vi "Add Subscription.vi"(8 "error in (no error)":errorcluster, 9 "SessionMailbox":refnum<queue>, 10 "Topic Subscription":T1, 11 "MQTT_Base in":refnum<class "MQTT_Base.lvclass">) -> (0 "error out":errorcluster, 1 "Failed":bool, 3 "MQTT_Base out":refnum<class "MQTT_Base.lvclass">)   [LabVIEW 2013, in "MQTT Base.lvlib" / "MQTT_Base.lvclass"]
uses:
  MQTT_Base.lvclass
  <vilib>/LabVIEW Open Source Project/MQTT Control Packets/Control Packets/SUBSCRIBE/Topic Subscription -- cluster.ctl
  <vilib>/LabVIEW Open Source Project/MQTT Control Packets/Control Packets/ControlPacket/QualityOfService -- enum.ctl
  Response -- cluster.ctl
  <vilib>/LabVIEW Open Source Project/MQTT Control Packets/Control Packets/ControlPacket/ControlPacket.lvclass
  MQTT_Base.lvclass/MQTT_Base.ctl
  Subscription/Subscription.lvclass/Subscription.ctl
  TopicFilter/TopicFilter.lvclass/TopicFilter.ctl
  Subscription/Subscription.lvclass
  <vilib>/LabVIEW Open Source Project/MQTT Control Packets/Control Packets/SUBSCRIBE/SUBSCRIBE.lvclass
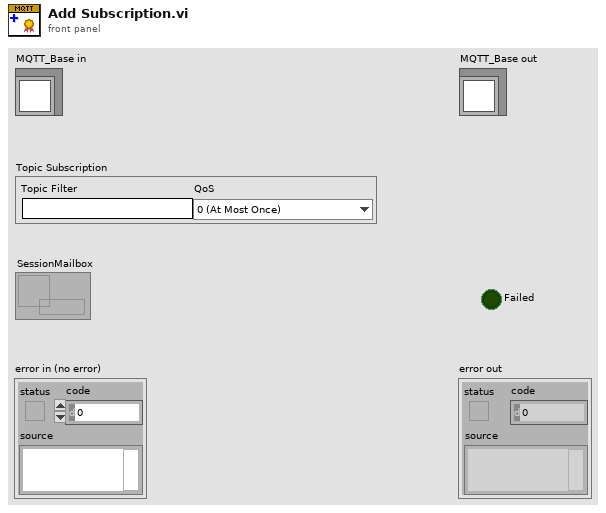
[diagram p1: front panel]
types:
  T1 = typedef "MQTT_Control_Packets.lvlib/SUBSCRIBE.lvclass/Topic Subscription -- cluster.ctl" = cluster{"Topic Filter":string, "QoS":T2}
  T2 = typedef "MQTT_Control_Packets.lvlib/ControlPacket.lvclass/QualityOfService -- enum.ctl" = enum16{"0 (At Most Once)", "1 (At Least Once)", "2 (Exactly Once)"}
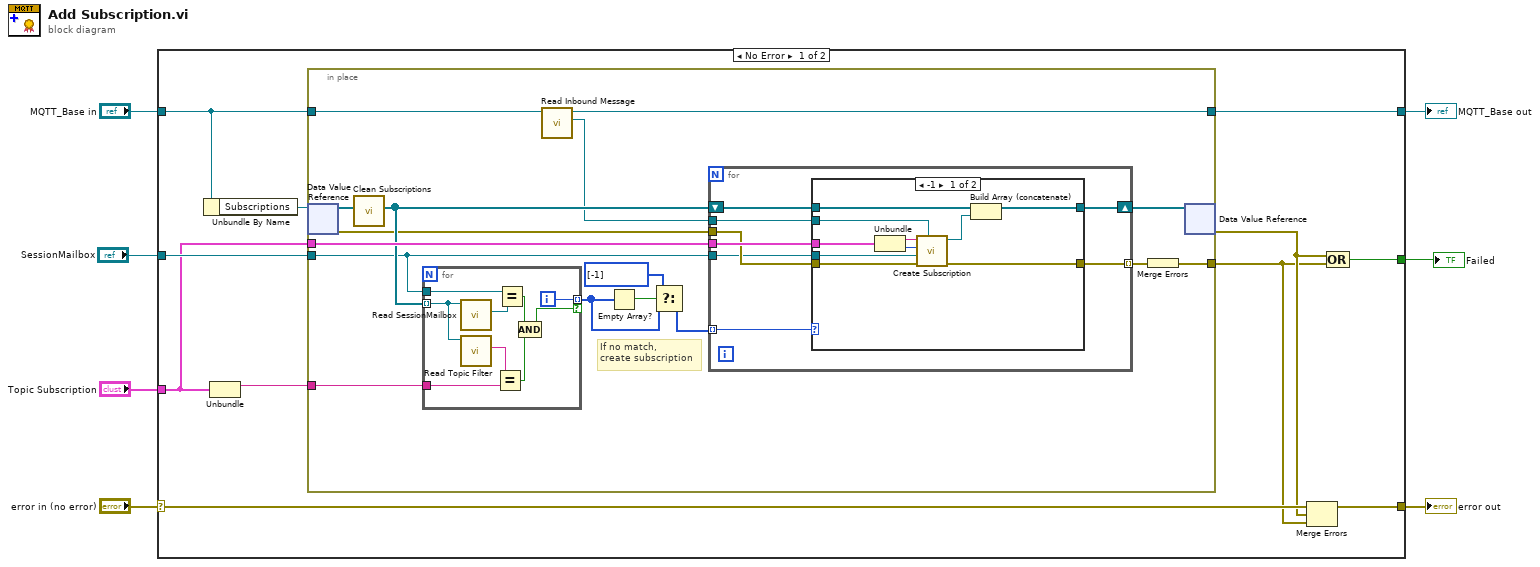
[diagram p0: block diagram]
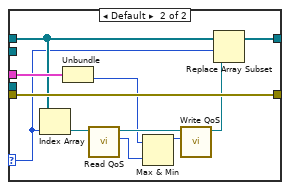
[diagram p2: hidden frame]
diagram:
  n1 = case shown="No Error" "error in (no error)" {
    selector: "error in (no error)" -> [w17 w74]
    tunnel: [w16 w74] -> w6
    tunnel: [w8 w73] -> w4
    tunnel: "MQTT_Base in" -> [w14 w73]
    tunnel: "Topic Subscription" -> [w12 _]
    tunnel: [w9 _] -> w2
    tunnel: "SessionMailbox" -> [w13 _]
    frame No Error {
      n2 = Unbundle By Name(w14) -> ("Subscriptions"=w18:refnum<data-value>)
      n3 = Unbundle(w12) -> ("Topic Filter"=w15:string)  [unwired: 1 out]
      n4 = in-place {
        in-place-border: w15 -> [w27]
        in-place-border: w14 -> [w26]
        in-place-border: w13 -> [w28]
        in-place-border: w12 -> [w33]
        in-place-border: [w24] -> w10
        in-place-border: [w23] -> w8
        # "If no match,\ncreate subscription"
        n5 = in-place-dvr #1(w18) -> (w31:refnum<class "Subscription.lvclass">[], w29:errorcluster)
        n6 = call "Clean Subscriptions.vi"("Subscriptions in"=w31) -> ("Subscriptions"=w30:refnum<class "Subscription.lvclass">[])  [unwired: 10 in]
        n7 = for {
          tunnel: w30 -> [w72] mode=indexing
          tunnel: w28 -> [w70]
          tunnel: w27 -> [w68]
          tunnel: [w65] -> w20 mode=indexing if=w64
          i -> [w65]
          n8 = call "Read SessionMailbox.vi"("Subscription in"=w72) -> ("SessionMailbox"=w71:refnum<queue>)  [unwired: 8 in, 2 out]
          n9 = call "Read Topic Filter.vi"("Subscription in"=w72) -> ("Topic Filter"=w69:string)  [unwired: 7 in, 3 out]
          n10 = Equal?(x=w69, y=w68) -> (x = y?=w66:bool)
          n11 = Equal?(x=w70, y=w71) -> (x = y?=w67:bool)
          n12 = Compound Arithmetic op=AND(w67, w66) -> (w64:bool)
        }
        n13 = call "Read Inbound Message.vi"("MQTT_Base in"=w26) -> ("Inbound Message"=w25:refnum<user-event>, "MQTT_Base out"=w23:refnum<class "MQTT_Base.lvclass">)  [unwired: 8 in, 1 out]
        n14 = Empty Array?(array=w20) -> (empty?=w22:bool)
        n15 = Select(t=i32[] [-1], s=w22, f=w20) -> (s? t:f=w21:i32[])
        n16 = for {
          tunnel: w33 -> [w41]
          tunnel: [w40] -> w32 mode=indexing
          tunnel: w29 -> [w38]
          tunnel: w28 -> [w37]
          shift-right: [w42] -> w34
          shift-left: w30 -> [w39]
          tunnel: w21 -> [w36] mode=indexing
          tunnel: w25 -> [w35]
          n17 = case shown="-1" w36 {
            selector: w36 -> [_ w59]
            tunnel: [w52 w62] -> w42
            tunnel: w39 -> [w51 w60]
            tunnel: w37 -> [w49 _]
            tunnel: w41 -> [w46 w63]
            tunnel: [w45 w61] -> w40
            tunnel: w38 -> [w44 w61]
            tunnel: w35 -> [w43 _]
            frame -1 {
              n18 = Unbundle(w46) -> ("Topic Filter"=w48:string, "QoS"=w47:T2)
              n19 = call "Create Subscription.vi"("Inbound Message"=w43, "error in (no error)"=w44, "SessionMailbox"=w49, "QoS"=w47, "Topic Filter"=w48) -> ("error out"=w45:errorcluster, "Subscription out"=w50:refnum<class "Subscription.lvclass">)  [unwired: 5 in]
              n20 = Build Array (concatenate)(w51, w50) -> (w52:refnum<class "Subscription.lvclass">[])
            }
            frame Default {
              n21 = Index Array(array=w60, index=w59) -> (element=w53:refnum<class "Subscription.lvclass">)
              n22 = Unbundle(w63) -> ("QoS"=w56:T2)  [unwired: 1 out]
              n23 = call "Read QoS.vi"("Subscription in"=w53) -> ("QoS"=w57:T2, "Subscription out"=w58:refnum<class "Subscription.lvclass">)  [unwired: 8 in, 1 out]
              n24 = Max & Min(x=w56, y=w57) -> (max(x,y)=w55:u16)  [unwired: 1 out]
              n25 = call "Write QoS.vi"("QoS"=w55, "Subscription in"=w58) -> ("Subscription out"=w54:refnum<class "Subscription.lvclass">)  [unwired: 8 in, 1 out]
              n26 = Replace Array Subset(array=w60, new element=w54, index=w59) -> (w62:refnum<class "Subscription.lvclass">[])
            }
          }
        }
        n27 = Merge Errors(w32) -> (w24:errorcluster)
        n28 = in-place-dvr #1(w34) -> (w11:errorcluster)  [unwired: 1 out]
      }
      n29 = Merge Errors(w17, w11, w10) -> (w16:errorcluster)
      n30 = Compound Arithmetic op=OR(w11, w10) -> (w9:bool)
    }
    frame Error {
    }
  }
  "error out" <- w6
  "MQTT_Base out" <- w4
  "Failed" <- w2
